vi "Milliseconds for Interval.vi"(10 "Interval":T1) -> (2 "Milliseconds":u32)   [LabVIEW 2021, in "Interval Timer.lvlib"]
doc: "Return the equivalent 'Milliseconds' for the input 'Interval'."
uses:
  Interval Timer.lvlib
  Interval Length.ctl
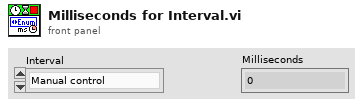
[diagram p1: front panel]
types:
  T1 = typedef "Interval Timer.lvlib/Interval Length.ctl" = enum16{"Manual control", "1 second", "10 seconds", "30 seconds", "60 seconds", "600 seconds", "1200 seconds", "3600 seconds"}
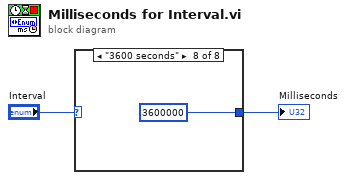
[diagram p0: block diagram]
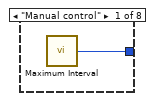
[diagram p2: hidden frame]
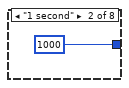
[diagram p3: hidden frame]
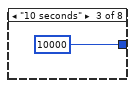
[diagram p4: hidden frame]
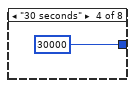
[diagram p5: hidden frame]
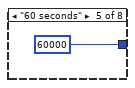
[diagram p6: hidden frame]
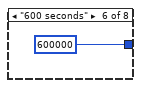
[diagram p7: hidden frame]
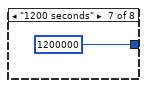
[diagram p8: hidden frame]
diagram:
  n1 = case shown="\"3600 seconds\"" "Interval" {
    tunnel: [w3 u32 1000 u32 10000 u32 30000 u32 60000 u32 600000 u32 1200000 u32 3600000] -> w1
    frame "Manual control" {
      n2 = call "Maximum Interval.vi"() -> ("New Acquisition Time"=w3:u32)
    }
    frame "1 second" {
    }
    frame "10 seconds" {
    }
    frame "30 seconds" {
    }
    frame "60 seconds" {
    }
    frame "600 seconds" {
    }
    frame "1200 seconds" {
    }
    frame "3600 seconds" {
    }
  }
  "Milliseconds" <- w1
